vi "DriveAngleHAdvanced.vi"(0 "Reinit":bool, 3 "Parameter String":string) -> (5 "Increment":bool, 7 "Error Out":errorcluster)   [LabVIEW 2019]
doc: "The swerve drive base will rotate about its center at a speed specified by the joystick command. This is a \"medium smart\" algorithm, the angle has to be within the specified range for a certain amount of time. Any complex or critical turns should be handled using either the Path Follower or auto-targeting. \n\nParameters:\n1. field-centric angle --> (deg) [0,360]\n2. error- the number of degrees on either side of the goal allowed --> (deg) [0,360]"
uses:
  SafeParser_Float.vi
  dsinstructions.vi
  sensors.vi
panel:
  in  "Time in Range (ms)":u32=1000
  in  "Plots?":bool
  out "Controller Summary":T1(graph)
  in  "PID Tuning Parameters":T2={"Kp"=0.01, "Ki"=0.01, "Kd"=9e-05, "N-Diff"=10, "N-Int"=20, "Int Error Window"=0.5, "Max Ouput"=1.0, "Min Output"=-1.0} {"Int Error Window" min=0.0; "N-Int" min=2; "N-Diff" min=2; "Kd" min=0.0; "Ki" min=0.0; "Kp" min=0.0}
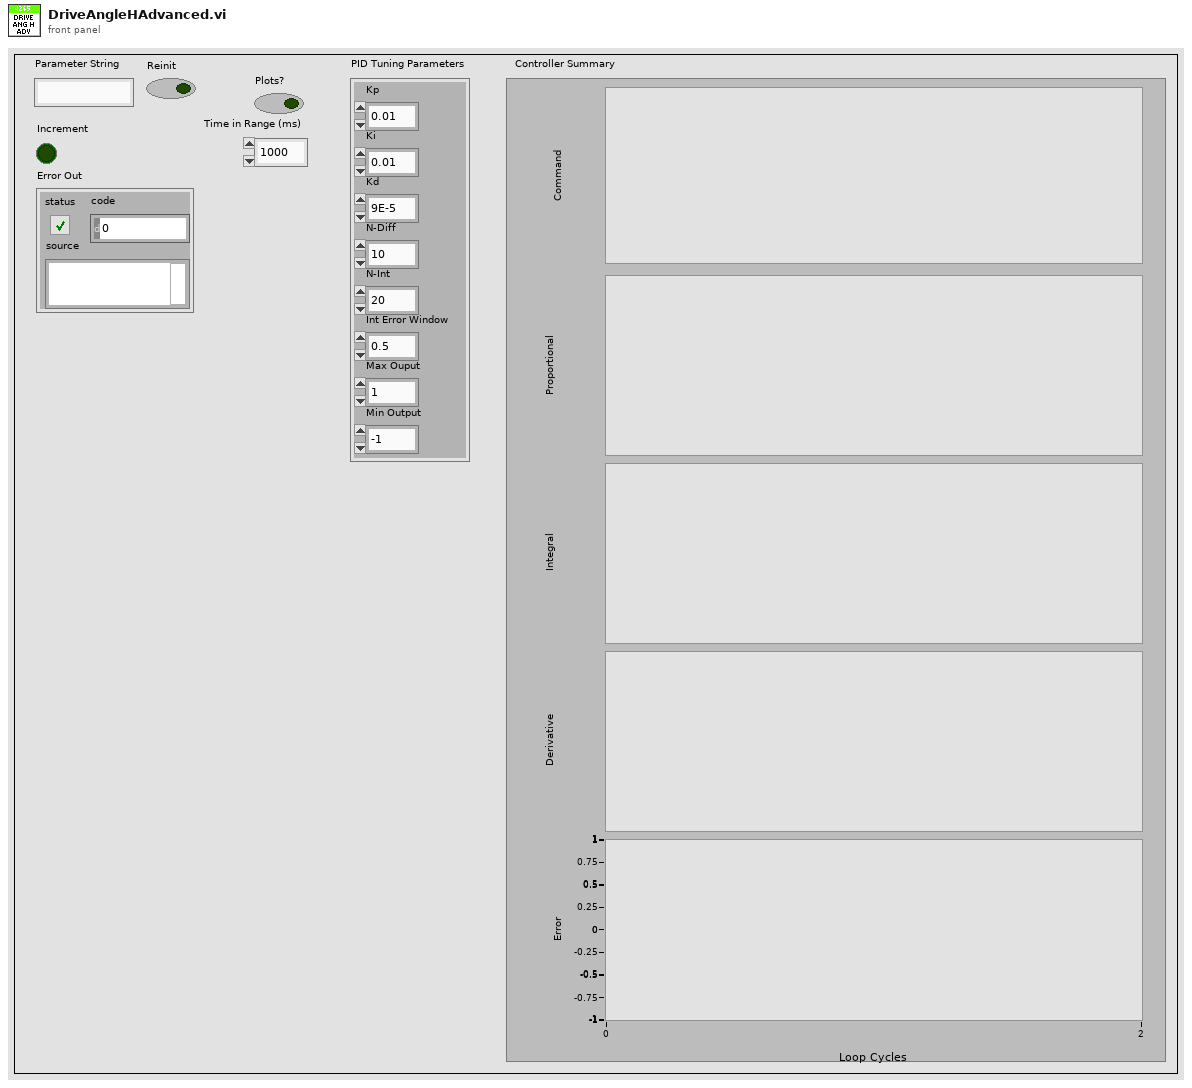
[diagram p1: front panel]
types:
  T1 = cluster{"Command":dbl, "Proportional":dbl, "Integral":dbl, "Derivative":dbl, "Goal":dbl}
  T2 = cluster{"Kp":dbl, "Ki":dbl, "Kd":dbl, "N-Diff":i32, "N-Int":i32, "Int Error Window":dbl, "Max Ouput":dbl, "Min Output":dbl}
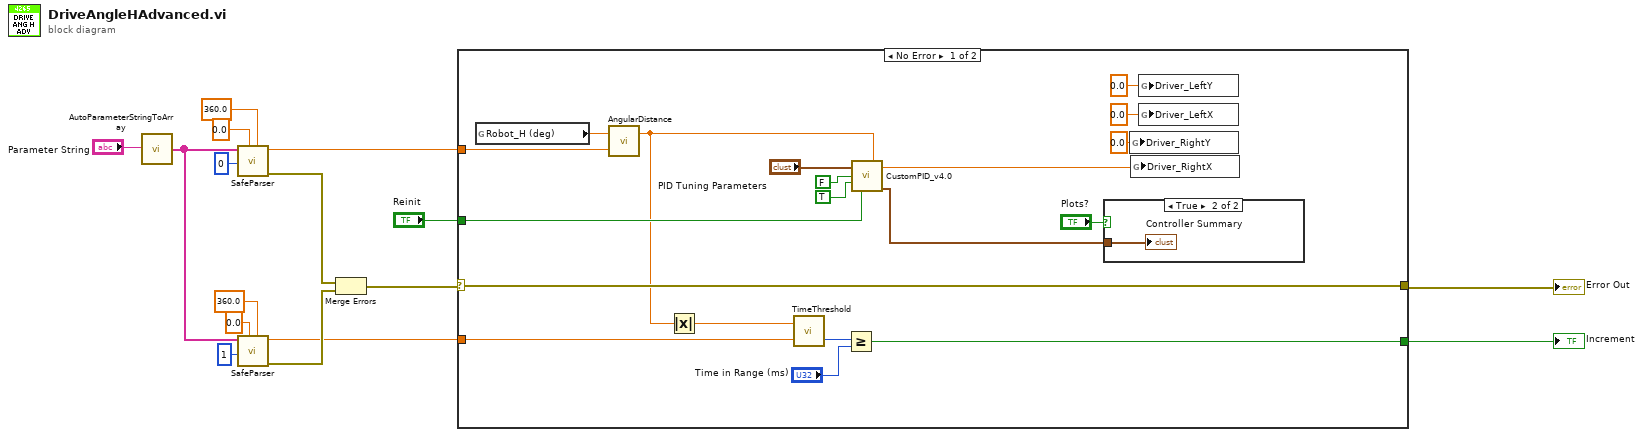
[diagram p0: block diagram]
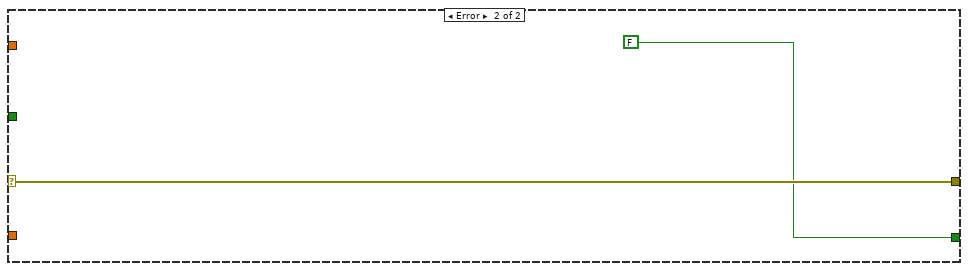
[diagram p3: hidden frame]
diagram:
  n1 = call "AutoParameterStringToArray.vi"("Parameter String"="Parameter String") -> ("Parsed Parameters"=w3:string[])
  n2 = call-poly "SafeParser.vi"("Maximum"=360.0, "Minimum"=0.0, "Array Index"=0 ("Parameter Index"), "String Array"=w3) -> ("Error Out"=w8:errorcluster, "Typecast  Value"=w6:dbl)  [unwired: 6 in]
  n3 = call-poly "SafeParser.vi"("Maximum"=360.0, "Minimum"=0.0, "Array Index"=1 ("Parameter Index"), "String Array"=w3) -> ("Error Out"=w7:errorcluster, "Typecast  Value"=w2:dbl)  [unwired: 6 in]
  n4 = Merge Errors(w8, w7) -> (w9:errorcluster)
  n5 = case shown="No Error" w9 {
    selector: w9 -> [w32 w38]
    tunnel: [w17 FALSE] -> w16
    tunnel: [w32 w38] -> w15
    tunnel: w6 -> [w31 _]
    tunnel: w2 -> [w18 _]
    tunnel: "Reinit" -> [w22 _]
    frame No Error {
      n6 = global read "sensors.vi" "Robot_H (deg)"() -> (w21:dbl)
      n7 = call "AngularDistance.vi"("Goal Angle (deg) [0,360]"=w31, "Current Angle (deg) [-Inf,+Inf]"=w21) -> ("Signed Angular Distance (deg) [-180,+180]"=w20:dbl)  [unwired: 1 out]
      n8 = Absolute Value(x=w20) -> (abs(x)=w19:dbl)
      n9 = call "TimeThreshold.vi"("Threshold"=w18, "Current Value"=w19) -> ("Time Below Threshold (ms)"=w24:u32)  [unwired: 1 out]
      n10 = Greater Or Equal?(x=w24, y="Time in Range (ms)") -> (x >= y?=w17:bool)
      n11 = call "CustomPID_v4.0.vi"("PID Tuning Parameters"="PID Tuning Parameters", "Custom Error Calculation"=w20, "Reset on Goal Change ?"=FALSE, "Use Custom Error Calculation ?"=TRUE ("Reset on Goal Change ?"), "Reinit"=w22) -> ("Command"=w27:dbl, "Controller Summary"=w25:T1)  [unwired: 7 in, 2 out]
      n12 = case shown="True" "Plots?" {
        tunnel: w25 -> [_ w36]
        frame False {
        }
        frame True {
          "Controller Summary" <- w36
        }
      }
      n13 = global write "dsinstructions.vi" "Driver_RightY"(0.0 ("Driver_RightX")) -> ()
      n14 = global write "dsinstructions.vi" "Driver_RightX"(w27) -> ()
      n15 = global write "dsinstructions.vi" "Driver_LeftY"(0.0 ("Driver_RightX")) -> ()
      n16 = global write "dsinstructions.vi" "Driver_LeftX"(0.0 ("Driver_RightX")) -> ()
    }
    frame Error {
    }
  }
  "Increment" <- w16
  "Error Out" <- w15
